vi "Get acquired data.vi"(8 "error in (no error)":errorcluster, 11 "CCD in":refnum<class "CCD.lvclass">) -> (0 "error out":errorcluster, 3 "CCD out":refnum<class "CCD.lvclass">)   [LabVIEW 2018, in "CCD.lvclass"]
uses:
  CCD.lvclass
  CCD.lvclass/CCD.ctl
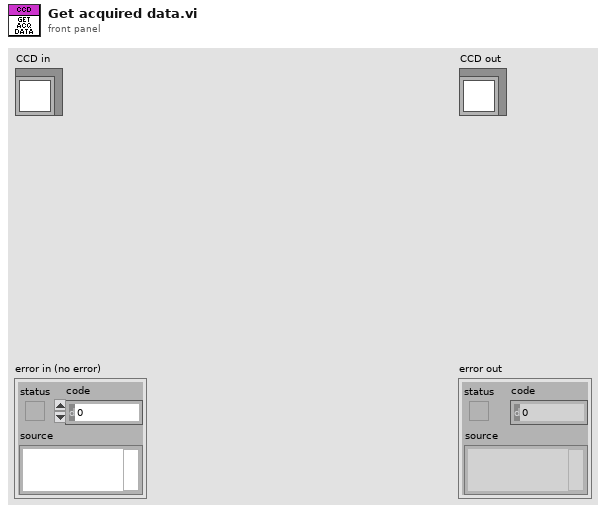
[diagram p1: front panel]
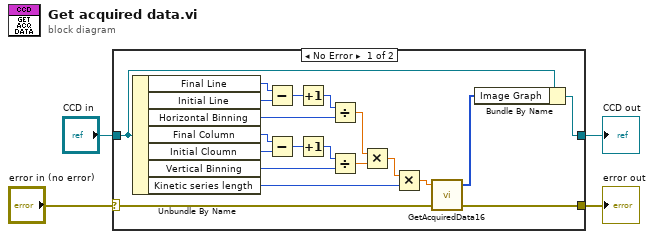
[diagram p0: block diagram]
diagram:
  n1 = case shown="No Error" "error in (no error)" {
    selector: "error in (no error)" -> [w7 w26]
    tunnel: [w8 w26] -> w2
    tunnel: [w24 w25] -> w1
    tunnel: "CCD in" -> [w11 w25]
    frame No Error {
      n2 = Unbundle By Name(w11) -> ("Final Line"=w23:u16, "Initial Line"=w22:u16, "Horizontal Binning"=w16:u16, "Final Column"=w21:u16, "Initial Cloumn"=w20:u16, "Vertical Binning"=w13:u16, "Kinetic series length"=w5:u32)
      n3 = Subtract(x=w23, y=w22) -> (x-y=w19:u16)
      n4 = Subtract(x=w21, y=w20) -> (x-y=w18:u16)
      n5 = Increment(x=w19) -> (x+1=w17:u16)
      n6 = Increment(x=w18) -> (x+1=w14:u16)
      n7 = Divide(x=w17, y=w16) -> (x/y=w15:dbl)
      n8 = Divide(x=w14, y=w13) -> (x/y=w12:dbl)
      n9 = Multiply(x=w15, y=w12) -> (x*y=w10:dbl)
      n10 = Multiply(x=w10, y=w5) -> (x*y=w9:dbl)
      n11 = call <userlib>:"GetAcquiredData16.vi"("error in (no error)"=w7, "size"=w9) -> ("error out"=w8:errorcluster, "array"=w6:u16[])  [unwired: 1 in, 1 out]
      n12 = Bundle By Name(cluster=w11, "Image Graph"=w6) -> (w24:refnum<class "CCD.lvclass">)
    }
    frame Error {
    }
  }
  "error out" <- w2
  "CCD out" <- w1
